vi "Write Resource Name.vi"(8 "error in (no error)":errorcluster, 10 "Resource Name":string, 11 "Chassis in":refnum<class "Chassis.lvclass">) -> (0 "error out":errorcluster, 3 "Chassis out":refnum<class "Chassis.lvclass">)   [LabVIEW 2015]
uses:
  Chassis.lvclass
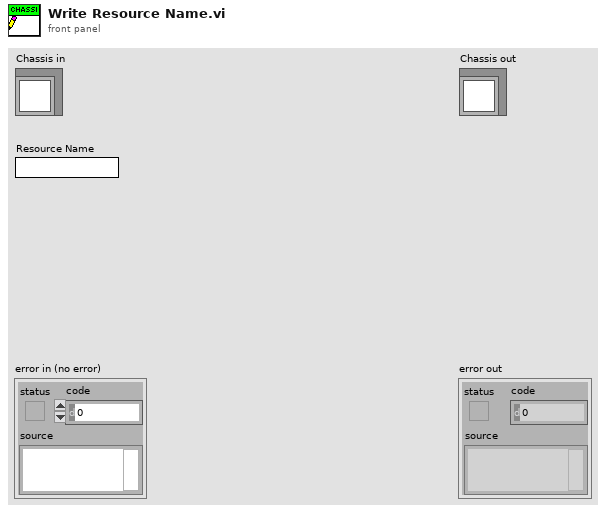
[diagram p1: front panel]
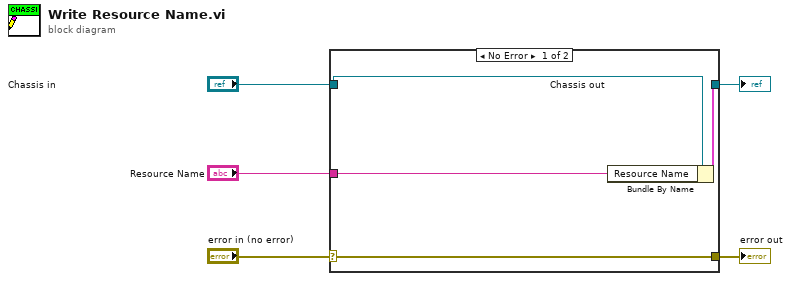
[diagram p0: block diagram]
diagram:
  n1 = case shown="No Error" "error in (no error)" {
    selector: "error in (no error)" -> [w9 w10]
    tunnel: [w9 w10] -> w4
    tunnel: [w7 w11] -> w2
    tunnel: "Chassis in" -> [w8 w11]
    tunnel: "Resource Name" -> [w6 _]
    frame No Error {
      n2 = Bundle By Name(cluster=w8, "Resource Name"=w6) -> (w7:cluster{})
    }
    frame Error {
    }
  }
  "error out" <- w4
  "Chassis out" <- w2
